vi "Write CSV File_2D (UTF-16).vi"(7 "delimiter (,) *ACSII":string=",", 8 "error in (no error)":errorcluster, 9 "append to file? (new file)":bool, 10 "2D array *UTF-16":string[][](array[string]), 11 "file path in":path) -> (0 "error out":errorcluster, 3 "file path out":path)   [LabVIEW 2013, in "SET_Robust CSV (UTF-16).lvlib"]
doc: "Write a 2D array of strings to CSV file. The CSV file is formatted in accordance with RFC-4180 (see http://tools.ietf.org/html/rfc4180). \n\nA custom delimiter character can be specified. Default is a comma.\n\nSetting \"append to file?\" to true will append the data to the end of an existing file. Setting \"append to file?\" to false will overwrite an existing file. In both cases, if the file is not found, a new file will be created.\n\nRev 0.0 2014-02-20 Ryan Porter\nFirst Draft"
uses:
  SET_Robust CSV (UTF-16).lvlib
panel:
  # "Write CSV File_2D.vi\n\nWrite a 2D array of strings to CSV file. The CSV file is formatted in accordance with RFC-4180 (see http://tools.ietf.org/html/rfc4180). \n\nA custom delimiter character can be specified. Default is a comma.\n\nSetting \"append to file?\" to true will append the data to the end of an existing file. Setting \"append to file?\" to false will overwrite an existing file. In both cases, if the file is not found, a new file will be created."
  # "License: BSD (2-Clause) - http://opensource.org/licenses/BSD-2-Clause \n\nCopyright (c) 2014, Ryan Porter\nAll rights reserved."
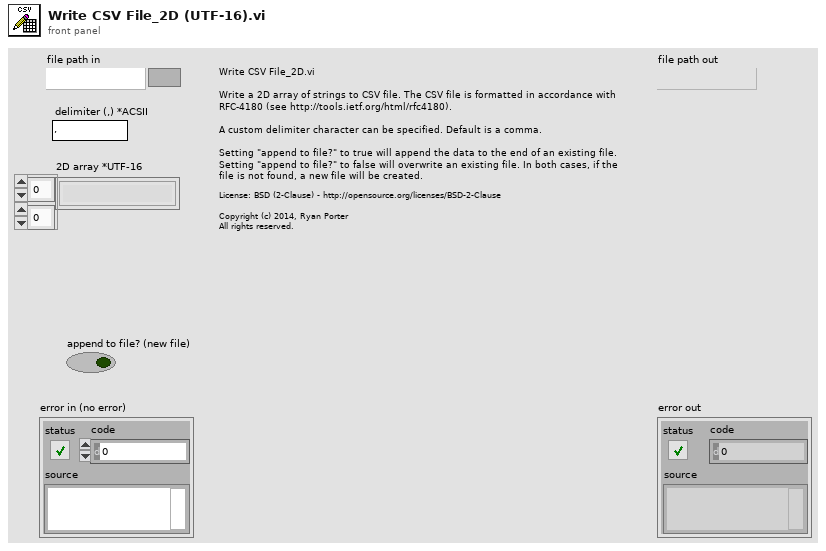
[diagram p1: front panel]
types:
  T1 = enum16{"open", "replace", "create", "open or create", "replace or create", "replace or create with confirmation"}
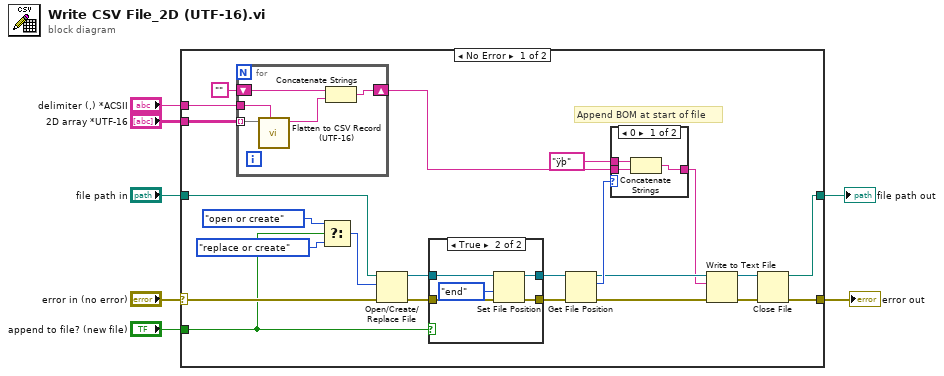
[diagram p0: block diagram]
diagram:
  n1 = case shown="No Error" "error in (no error)" {
    selector: "error in (no error)" -> [w27 w48]
    tunnel: "2D array *UTF-16" -> [w30 _]
    tunnel: "delimiter (,) *ACSII" -> [w28 _]
    tunnel: [w18 w48] -> w4
    tunnel: "file path in" -> [w26 w47]
    tunnel: "append to file? (new file)" -> [w20 _]
    tunnel: [w16 w47] -> w1
    frame No Error {
      # "Append BOM at start of file"
      n2 = for {
        tunnel: w30 -> [w44] mode=indexing
        shift-right: [w45] -> w10
        shift-left: "" -> [w46]
        tunnel: w28 -> [w43]
        n3 = call "Flatten to CSV Record (UTF-16).vi"("delimiter (,) *ASCII"=w43, "row of strings *UTF-16"=w44) -> ("CSV record *UTF-16"=w42:string)  [unwired: 8 in, 1 out]
        n4 = Concatenate Strings(w46, w42) -> (w45:string)
      }
      n5 = Select(t=T1."open or create" ("operation (0:open)"), s=w20, f=T1."replace or create" ("operation (0:open)")) -> (s? t:f=w23:T1)
      n6 = Open/Create/Replace File(file path (use dialog)=w26, error in=w27, operation (0:open)=w23) -> (refnum out=w22:refnum<file>, error out=w21:errorcluster)  [unwired: 3 in, 1 out]
      n7 = case shown="True" w20 {
        tunnel: w22 -> [w36 w41]
        tunnel: w21 -> [w35 w40]
        tunnel: [w35 w38] -> w8
        tunnel: [w36 w37] -> w9
        frame False {
        }
        frame True {
          n8 = Set File Position(refnum=w41, from (0:start)=enum16{"start", "end", "current"}."end", error in=w40) -> (refnum out=w37:refnum<file>, error out=w38:errorcluster)  [unwired: 1 in]
        }
      }
      n9 = Get File Position(4:w8, 7:w9) -> (0:w12:errorcluster, 2:w15:i64, 3:w13:refnum<file>)
      n10 = case shown="0" w15 {
        tunnel: w10 -> [w33 w34]
        tunnel: [w32 w34] -> w11
        tunnel: "ÿþ" -> [w31 _]
        frame 0 {
          n11 = Concatenate Strings(w31, w33) -> (w32:string)
        }
        frame 1, Default {
        }
      }
      n12 = Write to Text File(file (use dialog)=w13, text=w11, error in=w12) -> (refnum out=w17:refnum<file>, error out=w19:errorcluster)  [unwired: 1 in, 1 out]
      n13 = Close File(refnum=w17, error in=w19) -> (path=w16:path, error out=w18:errorcluster)
    }
    frame Error {
    }
  }
  "error out" <- w4
  "file path out" <- w1
